vi "Add Users.vi"(8 "error in (no error)":errorcluster, 10 "Users":refnum<class "User.lvclass">[](array[class]), 11 "InMemoryUserProvider in":refnum<class "InMemoryUserProvider.lvclass">) -> (0 "error out":errorcluster, 3 "InMemoryUserProvider out":refnum<class "InMemoryUserProvider.lvclass">)   [LabVIEW 2020, in "HTTP Server.lvlib" / "InMemoryUserProvider.lvclass"]
uses:
  InMemoryUserProvider.lvclass
  User/User.lvclass
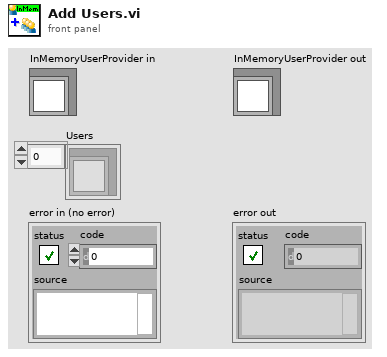
[diagram p1: front panel]
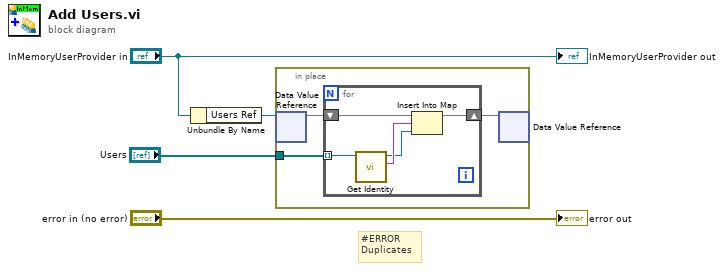
[diagram p0: block diagram]
diagram:
  # "#ERROR\nDuplicates"
  n1 = Unbundle By Name("InMemoryUserProvider in") -> ("Users Ref"=w3:refnum<data-value>)
  n2 = in-place {
    in-place-border: "Users" -> [w6]
    n3 = in-place-dvr #1(w3) -> (w7:map{string, refnum<class "User.lvclass">})  [unwired: 1 out]
    n4 = for {
      shift-right: [w8] -> w5
      shift-left: w7 -> [w11]
      tunnel: w6 -> [w12] mode=indexing
      n5 = call-dynamic "Get Identity.vi"("User in"=w12) -> ("Identity"=w10:string, "User out"=w9:refnum<class "User.lvclass">)  [unwired: 8 in, 1 out]
      n6 = Insert Into Map(map in=w11, key=w10, value=w9) -> (map out=w8:map{string, refnum<class "User.lvclass">})  [unwired: 2 out]
    }
    n7 = in-place-dvr #1(w5) -> ()  [unwired: 2 out]
  }
  "error out" <- "error in (no error)"
  "InMemoryUserProvider out" <- "InMemoryUserProvider in"
